vi "Actor Core.vi"(8 "error in":errorcluster, 11 "GUARDADOTEXTOPLANO in":refnum<class "GUARDADOTEXTOPLANO.lvclass">) -> (0 "error out":errorcluster, 3 "Actor out":refnum<class "Actor.lvclass">)   [LabVIEW 2019, in "GUARDADOTEXTOPLANO.lvlib" / "GUARDADOTEXTOPLANO.lvclass"]
doc: "(<B>Filename</B>: Actor Framework.lvlib:Actor.lvclass:Actor Core.vi)\n\nReceives messages to the actor, reacts to them, and initiates any error handling that may shut the actor down.\n\nDescendant classes may override this VI to append parallel tasks for the actor to complete while it handles messages. Overrides use the Call Parent Method node."
uses:
  GUARDADOTEXTOPLANO.lvclass
  <vilib>/ActorFramework/Actor/Actor.lvclass
  GUARDADOTEXTOPLANO.lvclass/GUARDADOTEXTOPLANO.ctl
panel:
  out "DATO":string
  out "PROVIENE DE?":enum16{"CONTADOR", "GENERADOR F"}(ring)
  out "Path":path
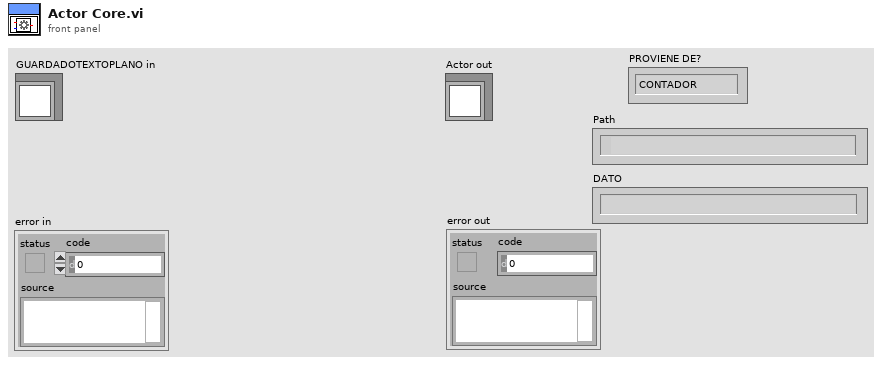
[diagram p1: front panel]
types:
  T1 = cluster{"Path":path, "PROVIENE DE?":enum16{"CONTADOR", "GENERADOR F"}, "DATO":string}
  T2 = cluster{"PATH":refnum<user-event>, "PROVIENE DE?":refnum<user-event>, "DATOS ":refnum<user-event>, "GUARDAR?":refnum<user-event>, "EXIT":refnum<user-event>}
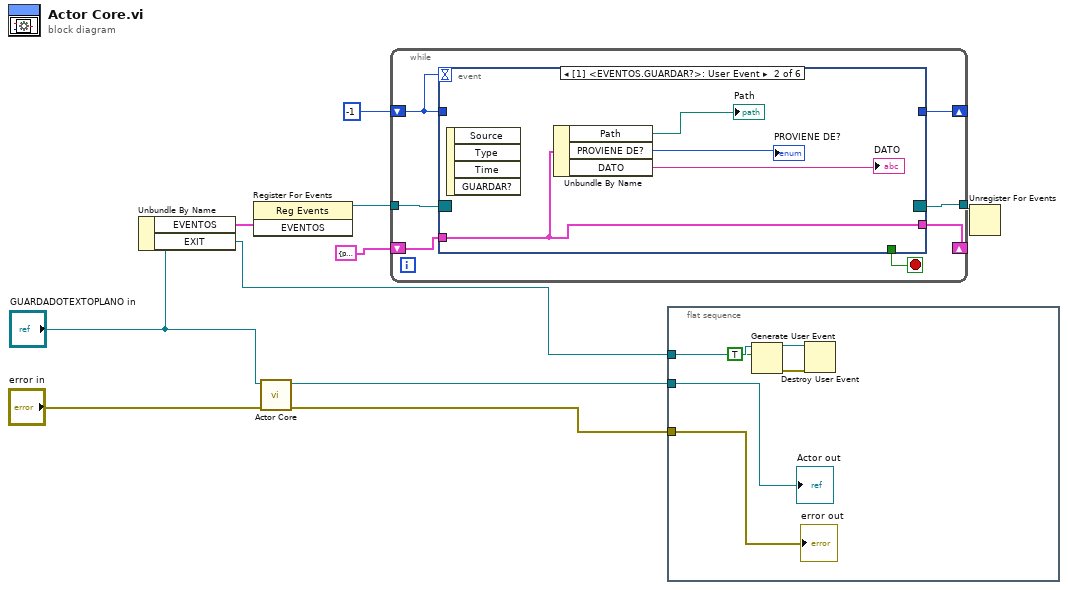
[diagram p0: block diagram]
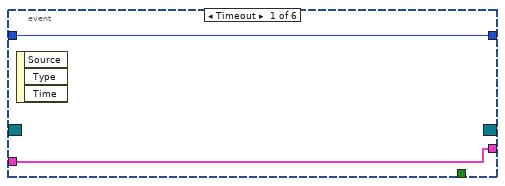
[diagram p2: hidden frame]
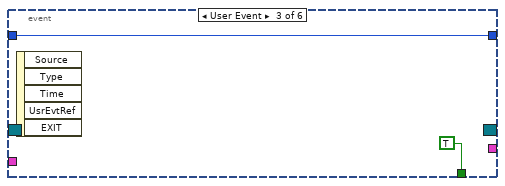
[diagram p3: hidden frame]
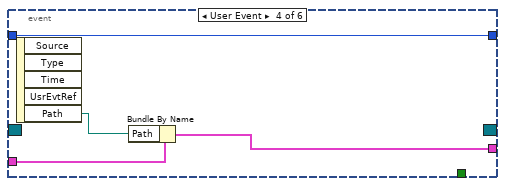
[diagram p4: hidden frame]
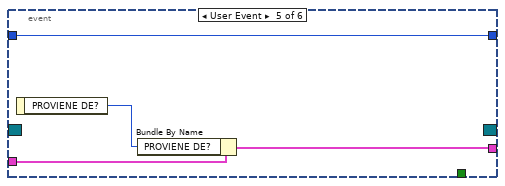
[diagram p5: hidden frame]
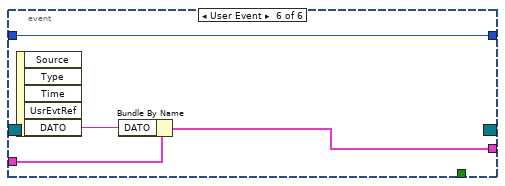
[diagram p6: hidden frame]
diagram:
  n1 = Unbundle By Name("GUARDADOTEXTOPLANO in") -> ("EVENTOS"=w6:T2, "EXIT"=w3:refnum<user-event>)
  n2 = register-events(w6) -> (reference out=w5:refnum<event-registration>)  [unwired: 2 in, 1 out]
  n3 = call-parent "Actor Core.vi"("error in"="error in", "Actor in"="GUARDADOTEXTOPLANO in") -> ("error out"=w10:errorcluster, "Actor out"=w9:refnum<class "Actor.lvclass">)  [unwired: 8 in]
  n4 = while {
    tunnel: w5 -> [w17]
    tunnel: [w16] -> w4
    shift-right: [w14] -> _
    shift-left: -1 -> [w15]
    shift-right: [w11] -> _
    shift-left: T1 {"Path"=path "", "PROVIENE DE?"=enum."CONTADOR", "DATO"=""} -> [w12]
    stop <- w13 stop-if-true
    n5 = event shown="[1] <EVENTOS.GUARDAR?>: User Event" {
      selector: w17 -> [_ _ _ _ _ _]
      dyn-events: [_ _ _ _ _ _] -> w16
      timeout: w15 -> [_ _ _ _ _ _]
      tunnel: w15 -> [w19 _ w24 w26 w30 w34]
      tunnel: [w19 _ w24 w26 w30 w34] -> w14
      tunnel: [_ _ TRUE _ _ _] -> w13
      tunnel: w12 -> [w18 w20 _ w29 w33 w37]
      tunnel: [w18 w20 _ w28 w32 w36] -> w11
      event Timeout {
        n6 = event-data() -> ()  [unwired: 1 in, 3 out]
      }
      event User Event {
        n7 = event-data() -> ()  [unwired: 1 in, 4 out]
        n8 = Unbundle By Name(w20) -> ("Path"=→"Path":path, "PROVIENE DE?"=→"PROVIENE DE?":enum16{"CONTADOR", "GENERADOR F"}, "DATO"=→"DATO":string)
      }
      event User Event {
        n9 = event-data() -> ()  [unwired: 1 in, 5 out]
      }
      event User Event {
        n10 = event-data() -> ("Path"=w27:path)  [unwired: 1 in, 4 out]
        n11 = Bundle By Name(cluster=w29, "Path"=w27) -> (w28:T1)
      }
      event User Event {
        n12 = event-data() -> ("PROVIENE DE?"=w31:enum16{"CONTADOR", "GENERADOR F"})  [unwired: 1 in]
        n13 = Bundle By Name(cluster=w33, "PROVIENE DE?"=w31) -> (w32:T1)
      }
      event User Event {
        n14 = event-data() -> ("DATO"=w35:string)  [unwired: 1 in, 4 out]
        n15 = Bundle By Name(cluster=w37, "DATO"=w35) -> (w36:T1)
      }
    }
  }
  n16 = flat-sequence {
    tunnel: w10 -> [w43]
    tunnel: w9 -> [w42]
    tunnel: w3 -> [w41]
    frame #0 {
      n17 = Generate User Event(user event=w41, event data cluster=TRUE ("event data")) -> (user event out=w38:refnum<user-event>, error out=w39:errorcluster)  [unwired: 2 in]
      n18 = Destroy User Event(user event=w38, error in=w39) -> ()  [unwired: 1 out]
      "error out" <- w43
      "Actor out" <- w42
    }
  }
  n19 = Unregister For Events(event registration refnum=w4) -> ()  [unwired: 1 in, 1 out]
